vi "Fit Result to String.vi"(8 "error in (no error)":errorcluster, 11 "Mean Fit in":refnum<class "Mean Fit.lvclass">) -> (0 "error out":errorcluster, 2 "Array":string[](array[string]), 3 "Mean Fit out":refnum<class "Mean Fit.lvclass">)   [LabVIEW 2013, in "Mean Fit.lvclass"]
uses:
  Mean Fit.lvclass
  Mean Fit.lvclass/Mean Fit.ctl
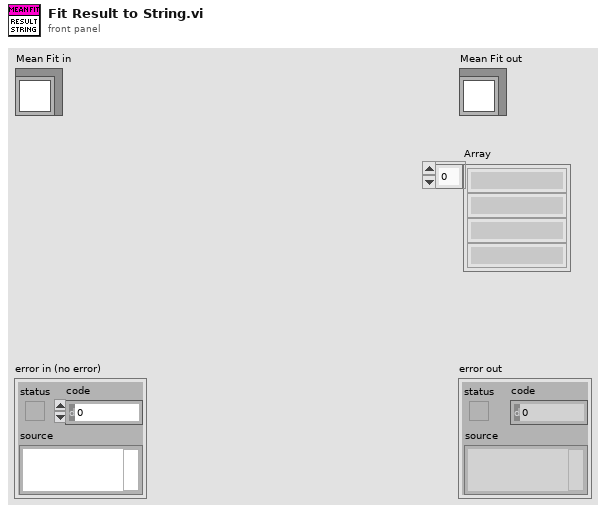
[diagram p1: front panel]
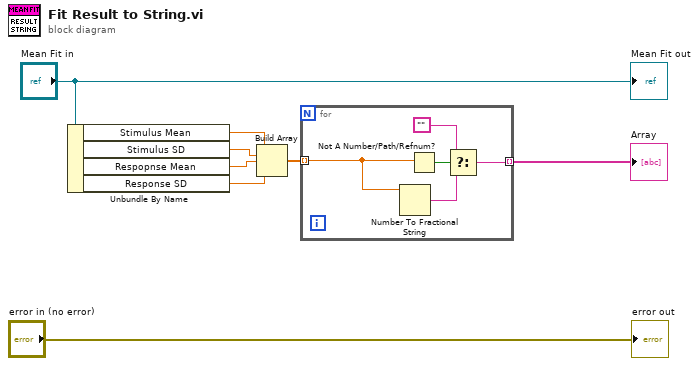
[diagram p0: block diagram]
diagram:
  n1 = Unbundle By Name("Mean Fit in") -> ("Stimulus Mean"=w6:dbl, "Stimulus SD"=w5:dbl, "Respopnse Mean"=w4:dbl, "Response SD"=w3:dbl)
  n2 = Build Array(w6, w5, w4, w3) -> (w2:dbl[])
  n3 = for {
    tunnel: [w13] -> w1 mode=indexing
    tunnel: w2 -> [w9] mode=indexing
    n4 = Number To Fractional String(number=w9) -> (F-format string=w10:string)  [unwired: 3 in]
    n5 = Not A Number/Path/Refnum?(number/path/refnum=w9) -> (NaN/Path/Refnum?=w12:bool)
    n6 = Select(t="", s=w12, f=w10) -> (s? t:f=w13:string)
  }
  "Array" <- w1
  "error out" <- "error in (no error)"
  "Mean Fit out" <- "Mean Fit in"
